vi "Display Console View.vi"(8 "error in (no error)":errorcluster, 11 "View Model":T2) -> (0 "error out":errorcluster)   [LabVIEW 2013]
doc: "Display console for debugging elevator operation."
uses:
  View Model/Controls/View Model.ctl
  Error/Controls/Error Model.ctl
  Error/Controls/Error Types.ctl
  View Model/Controls/Shared Model.ctl
  Elevator Controller/Controls/Elevator Model.ctl
  Elevator Controller/Controls/Controller Overhead.ctl
  Elevator Controller/Controls/Elevator States.ctl
  Elevator Controller/Controls/Elevator Location.ctl
  Elevator Controller/Controls/Elevator Command Event.ctl
  Elevator Controller/Controls/Elevator Commands.ctl
  Configuration/Controls/Configuration Model.ctl
  Configuration/Controls/Configuration Data.ctl
panel:
  out "Emergency":bool
  out "Door Open":bool
  out "Down":bool
  out "Up":bool
  out "Elevator Location":T1
  out "Timing":dbl
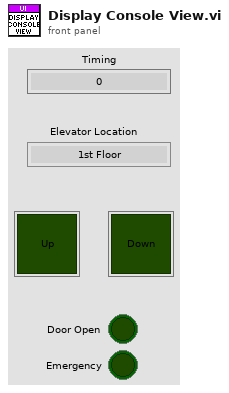
[diagram p1: front panel]
types:
  T1 = typedef "Elevator Location.ctl" = enum16{"1st Floor", "2nd Floor", "3rd Floor", "4th Floor"}
  T2 = typedef "View Model.ctl" = cluster{"Error Model":T3, "Shared Model":T4, "Elevator Model":T5, "Configuration Model":T6}
  T3 = typedef "Error Model.ctl" = cluster{"Error Event":refnum<user-event>}
  T4 = typedef "Shared Model.ctl" = cluster{"Stop DVR":refnum<data-value>, "Stop Event":refnum<user-event>}
  T5 = typedef "Elevator Model.ctl" = cluster{"Controller Overhead":refnum<data-value>, "Motion Change":refnum<user-event>, "Direction Change":refnum<user-event>, "Door Position Change":refnum<user-event>, "Emergency Change":refnum<user-event>, "Floor Change":refnum<user-event>, "Elevator Cmd":refnum<user-event>}
  T6 = typedef "Configuration Model.ctl" = cluster{"Configuration":refnum<data-value>, "Config Change":refnum<user-event>}
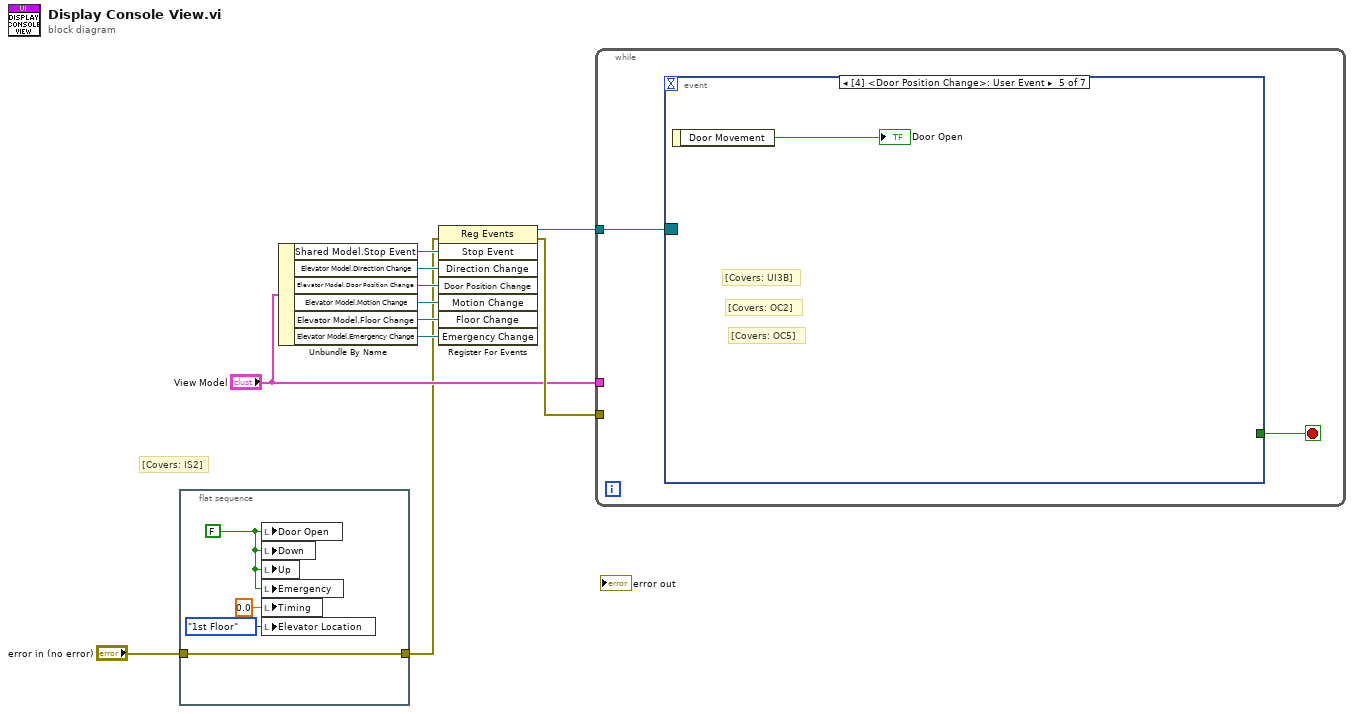
[diagram p0: block diagram]
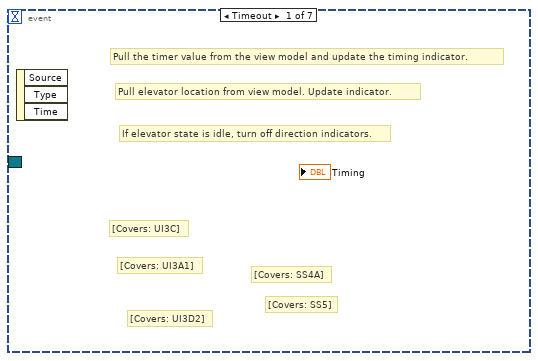
[diagram p2: hidden frame]
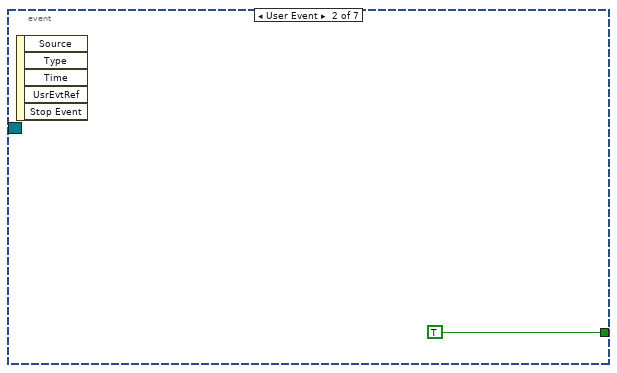
[diagram p3: hidden frame]
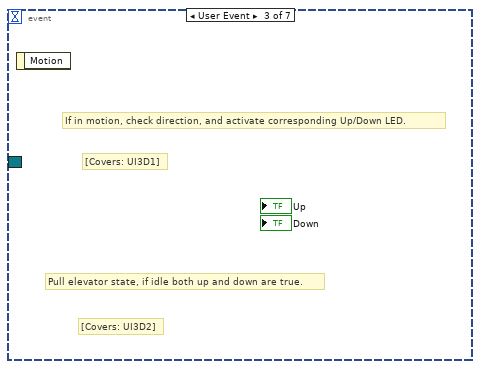
[diagram p4: hidden frame]
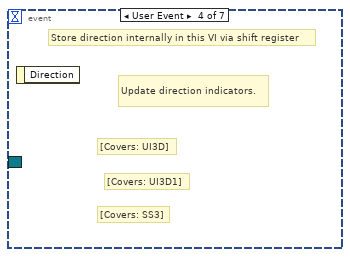
[diagram p5: hidden frame]
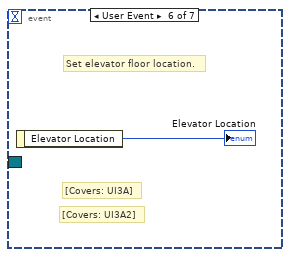
[diagram p6: hidden frame]
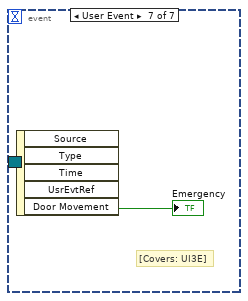
[diagram p7: hidden frame]
diagram:
  # "[Covers: IS2]"
  n1 = flat-sequence {
    tunnel: "error in (no error)" -> [w12]
    tunnel: [w12] -> w1
    frame #0 {
      w15 = FALSE ("Door Open")
      n2 = local write "Door Open"(w15) -> ()
      n3 = local write "Down"(w15) -> ()
      n4 = local write "Up"(w15) -> ()
      n5 = local write "Emergency"(w15) -> ()
      n6 = local write "Timing"(0.0 ("Timing")) -> ()
      n7 = local write "Elevator Location"(Elevator_Location."1st Floor" ("Elevator Location")) -> ()
    }
  }
  n8 = Unbundle By Name("View Model") -> ("Shared Model.Stop Event"=w8:refnum<user-event>, "Elevator Model.Direction Change"=w9:refnum<user-event>, "Elevator Model.Door Position Change"=w10:refnum<user-event>, "Elevator Model.Motion Change"=w11:refnum<user-event>, "Elevator Model.Floor Change"=w4:refnum<user-event>, "Elevator Model.Emergency Change"=w3:refnum<user-event>)
  n9 = register-events(error in=w1, w8, w9, w10, w11, w4, w3) -> (reference out=w7:refnum<event-registration>, error out=w6:errorcluster)  [unwired: 1 in]
  n10 = while {
    tunnel: w7 -> [w17]
    tunnel: w6 -> [_]
    tunnel: "View Model" -> [_]
    stop <- w16 stop-if-true
    n11 = event shown="[4] <Door Position Change>: User Event" {
      selector: w17 -> [_ _ _ _ _ _ _]
      dyn-events: _ -> [_ _ _ _ _ _ _]
      timeout: _ -> [_ _ _ _ _ _ _]
      tunnel: [_ TRUE _ _ _ _ _] -> w16
      event Timeout {
        # "[Covers: SS5]"
        # "[Covers: SS4A]"
        # "[Covers: UI3D2]"
        # "If elevator state is idle, turn off direction indicators."
        # "[Covers: UI3A1]"
        # "Pull elevator location from view model. Update indicator."
        # "[Covers: UI3C]"
        # "Pull the timer value from the view model and update the timing indicator."
        n12 = event-data() -> ()  [unwired: 1 in, 3 out]
      }
      event User Event {
        n13 = event-data() -> ()  [unwired: 1 in, 5 out]
      }
      event User Event {
        # "[Covers: UI3D2]"
        # "Pull elevator state, if idle both up and down are true."
        # "[Covers: UI3D1]"
        # "If in motion, check direction, and activate corresponding Up/Down LED."
        n14 = event-data() -> ()  [unwired: 1 in, 1 out]
      }
      event User Event {
        # "[Covers: SS3]"
        # "[Covers: UI3D1]"
        # "Update direction indicators."
        # "[Covers: UI3D]"
        # "Store direction internally in this VI via shift register"
        n15 = event-data() -> ()  [unwired: 1 in, 1 out]
      }
      event User Event {
        # "[Covers: OC5]"
        # "[Covers: OC2]"
        # "[Covers: UI3B]"
        n16 = event-data() -> ("Door Movement"=→"Door Open":bool)  [unwired: 1 in]
      }
      event User Event {
        # "[Covers: UI3A2]"
        # "[Covers: UI3A]"
        # "Set elevator floor location."
        n17 = event-data() -> ("Elevator Location"=→"Elevator Location":T1)  [unwired: 1 in]
      }
      event User Event {
        # "[Covers: UI3E]"
        n18 = event-data() -> ("Door Movement"=→"Emergency":bool)  [unwired: 1 in, 4 out]
      }
    }
  }
